vi "Ref Display.vi"(5 "Offset":refnum<class "Offset.lvclass"> caption="Offset (Cascade)", 6 "Size":refnum<class "Size.lvclass"> caption="Size (Unchanged)", 7 "Alignment":T1 caption="Alignment (Left, Top)", 8 "Error In":errorcluster, 10 "Display (Primary)":i32=-1) -> (0 "Error Out":errorcluster, 3 "Ref Display out":refnum<class "Ref Display.lvclass">)   [LabVIEW 2023, in "Panel Actor.lvlib" / "Panel.lvlib" / "Ref Display.lvclass"]
doc: "Positions a window with respect to a display.\n\n<B>Display:</B> Sets the display to use.\n<B>Alignment:</B> Set the type of alignment\n<B>Offset:</B> Input Offset object.\n<B>Size:</B> Display Size object.\n<B>Error In:</B> Describes error conditions that occur before this node runs.\n\n<B>Ref Display Out:</B> Reference Display object.\n<B>Error Out:</B> Contains error information.\n----\nPlease see the following web address for additional documentation and tutorial information:\nhttp://www.mooregoodideas.com/mgi-panel-manager/\n\nAuthor: Derek Trepanier\n\nCopyright (c) 2018, Moore Good Ideas, Inc.\n\nAll rights reserved.\n\nRedistribution and use in source and binary forms, with or without modification, are permitted provided that the following conditions are met:\n\n * Redistributions of source code must retain the above copyright notice, this list of conditions and the following disclaimer.\n * Redistributions in binary form must reproduce the above copyright notice, this list of conditions and the following disclaimer in the documentation and/or other materials provided with the distribution.\n * Neither the name of Moore Good Ideas, Inc. nor the names of its contributors may be used to endorse or promote products derived from this software without specific prior written permission.\n\nTHIS SOFTWARE IS PROVIDED BY THE COPYRIGHT HOLDERS AND CONTRIBUTORS \"AS IS\" AND ANY EXPRESS OR IMPLIED WARRANTIES, INCLUDING, BUT NOT LIMITED TO, THE IMPLIED WARRANTIES OF MERCHANTABILITY AND FITNESS FOR A PARTICULAR PURPOSE ARE DISCLAIMED. IN NO EVENT SHALL THE COPYRIGHT OWNER OR CONTRIBUTORS BE LIABLE FOR ANY DIRECT, INDIRECT, INCIDENTAL, SPECIAL, EXEMPLARY, OR CONSEQUENTIAL DAMAGES (INCLUDING, BUT NOT LIMITED TO, PROCUREMENT OF SUBSTITUTE GOODS OR SERVICES; LOSS OF USE, DATA, OR PROFITS; OR BUSINESS INTERRUPTION) HOWEVER CAUSED AND ON ANY THEORY OF LIABILITY, WHETHER IN CONTRACT, STRICT LIABILITY, OR TORT (INCLUDING NEGLIGENCE OR OTHERWISE) ARISING IN ANY WAY OUT OF THE USE OF THIS SOFTWARE, EVEN IF ADVISED OF THE POSSIBILITY OF SUCH DAMAGE."
uses:
  Ref Display.lvclass
  Offset/Offset.lvclass
  Alignment.ctl
  Horizontal Alignment.ctl
  Vertical Alignment.ctl
  Size/Size.lvclass
  Offset/Cascade/Cascade.lvclass/Cascade.ctl
  Ref Display.lvclass/Ref Display.ctl
  Offset/Cascade/Cascade.lvclass
  Reference Position.lvclass
  C:/Users/Public/Documents/Development/Engine/Panel Manager/Panel/Window Position/Reference Position/Offset/Offset.lvclass
  C:/Users/Public/Documents/Development/Engine/Panel Manager/Panel/Window Position/Reference Position/Offset/Cascade/Cascade.lvclass
  C:/Users/Public/Documents/Development/Engine/Panel Manager/Panel/Window Position/Reference Position/Reference Position.lvclass
  C:/Users/Public/Documents/Development/Engine/Panel Manager/Panel/Window Position/Window Position.lvclass
  C:/Users/Public/Documents/Development/Engine/Panel Manager/Panel/Window Position/Reference Position/Ref Display/Ref Display.lvclass
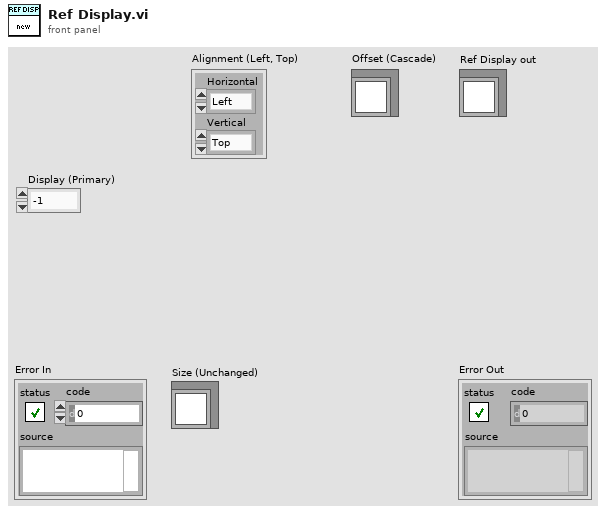
[diagram p1: front panel]
types:
  T1 = typedef "Panel Actor.lvlib/Panel.lvlib/Reference Position.lvclass/Alignment.ctl" = cluster{"Horizontal":T2, "Vertical":T3}
  T2 = typedef "Panel Actor.lvlib/Panel.lvlib/Reference Position.lvclass/Horizontal Alignment.ctl" = enum16{"Left", "Center", "Right"}
  T3 = typedef "Panel Actor.lvlib/Panel.lvlib/Reference Position.lvclass/Vertical Alignment.ctl" = enum16{"Top", "Center", "Bottom"}
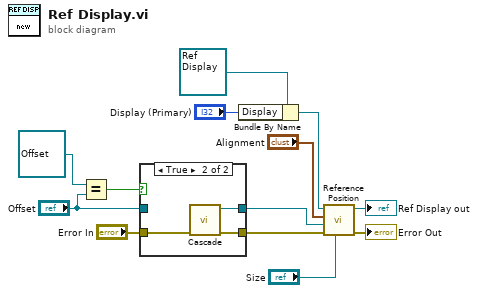
[diagram p0: block diagram]
diagram:
  n1 = Equal?(x=refnum<class "Offset.lvclass"> refnum ("y"), y="Offset") -> (x = y?=w7:bool)
  n2 = case shown="True" w7 {
    tunnel: "Error In" -> [w14 w18]
    tunnel: [w14 w17] -> w5
    tunnel: [w15 w16] -> w3
    tunnel: "Offset" -> [w15 _]
    frame False {
    }
    frame True {
      n3 = call "Cascade.vi"("Error In"=w18) -> ("Error Out"=w17:errorcluster, "Cascade out"=w16:refnum<class "Cascade.lvclass">)  [unwired: 9 in]
    }
  }
  n4 = Bundle By Name(cluster=refnum<class "Ref Display.lvclass"> refnum ("Ref Display in"), "Display"="Display (Primary)") -> (w11:refnum<class "Ref Display.lvclass">)
  n5 = call "Reference Position.vi"("Size"="Size", "error in (no error)"=w5, "Offset"=w3, "Alignment"="Alignment", "Reference Position in"=w11) -> ("error out"=→"Error Out":errorcluster, "Reference Position in"=→"Ref Display out":refnum<class "Ref Display.lvclass">)  [unwired: 5 in]
